vi "SR860 Ramp DC+AC Voltage.vi"() -> ()   [LabVIEW 2025]
doc: "VI to ramp DC Offset of SR860/865 Lockin over time. AC amplitude is kept constant.\nFor I-V curves\nScott Hannahs NHMFL <sth@magnet.fsu.edu>\nAuthor: Scott Hannahs <sth@magnet.fsu.edu>\n\nThis software is licensed for use under the “MIT License\"\nCopyright (c) 2025 Scott Hannahs, sth@sth@magnet.sthnet.net\n\nPermission is hereby granted, free of charge, to any person obtaining a copy of this software and associated documentation files (the \"Software\"), to deal in the Software without restriction, including without limitation the rights to use, copy, modify, merge, publish, distribute, sublicense, and/or sell copies of the Software, and to permit persons to whom the Software is furnished to do so, subject to the following conditions: The above copyright notice and this permission notice shall be included in all copies or substantial portions of the Software.\n\nTHE SOFTWARE IS PROVIDED \"AS IS\", WITHOUT WARRANTY OF ANY KIND, EXPRESS OR IMPLIED, INCLUDING BUT NOT LIMITED TO THE WARRANTIES OF MERCHANTABILITY, FITNESS FOR A PARTICULAR PURPOSE AND NONINFRINGEMENT. IN NO EVENT SHALL THE AUTHORS OR COPYRIGHT HOLDERS BE LIABLE FOR ANY CLAIM, DAMAGES OR OTHER LIABILITY, WHETHER IN AN ACTION OF CONTRACT, TORT OR OTHERWISE, ARISING FROM, OUT OF OR IN CONNECTION WITH THE SOFTWARE OR THE USE OR OTHER DEALINGS IN THE SOFTWARE."
panel:
  in  "AC Voltage":dbl=1e-09 min=1e-09 max=2.0 format="%.6g"
  in  "Clone":bool
  out "Time Remaining":dbl=60.0 format="%<%H:%M:%S>t"
  out "DC Output Voltage":dbl format="%_7g"
  in  "Time (Hr:Min:Sec)":dbl=60.0 step=1.0 format="%<%H:%M:%S>t"
  in  "DC Stop Voltage":dbl min=-5.0 max=5.0 format="%.6g"
  in  "Start Ramp":bool
  in  "Update Time":dbl=0.1 format="%.3g"
  in  "stop":bool
  in  "VISA resource name":refnum<visa-resource-name>
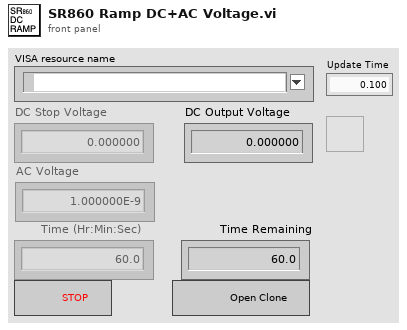
[diagram p1: front panel]
types:
  T1 = enum8{"Enabled", "Disabled", "Disabled and Grayed Out"}
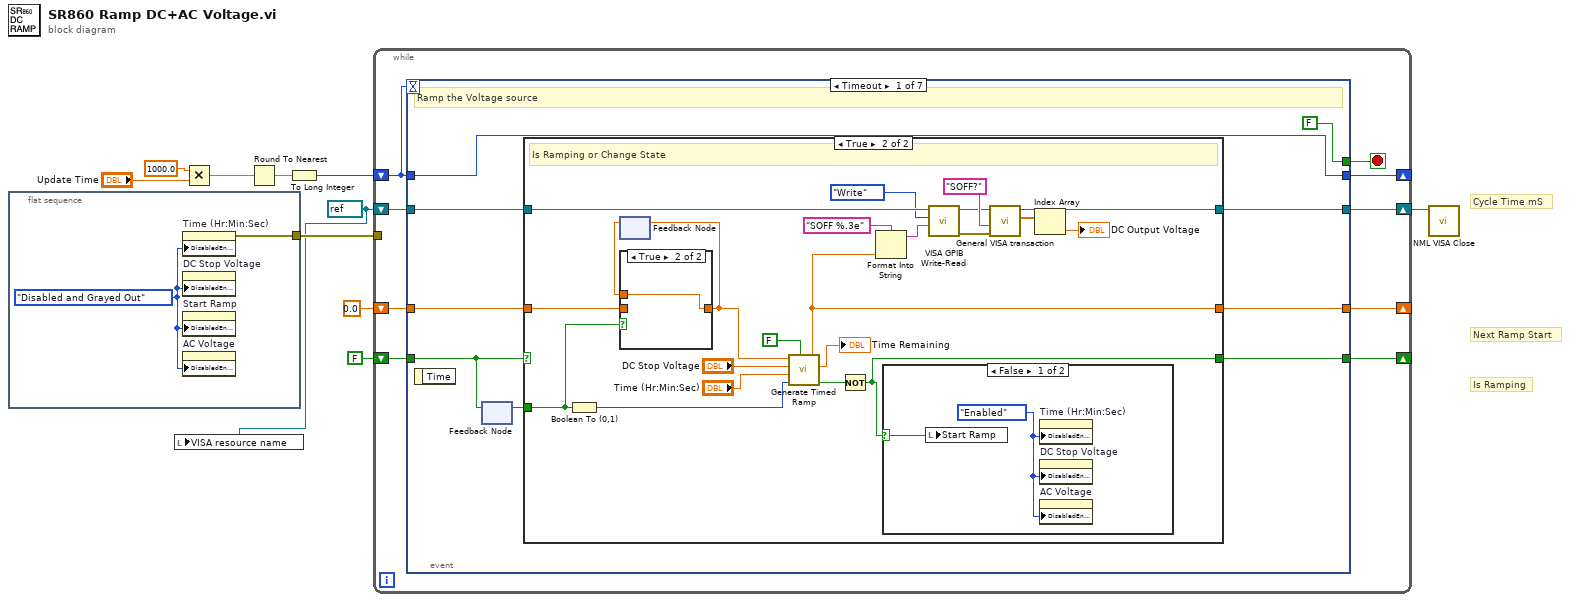
[diagram p0: block diagram]
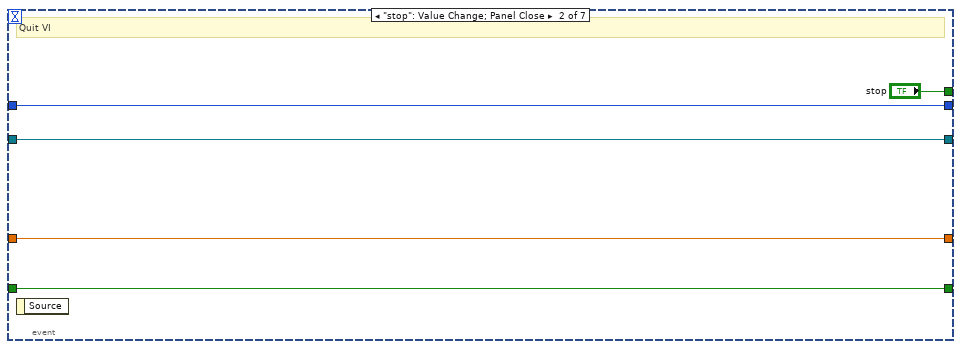
[diagram p5: hidden frame]
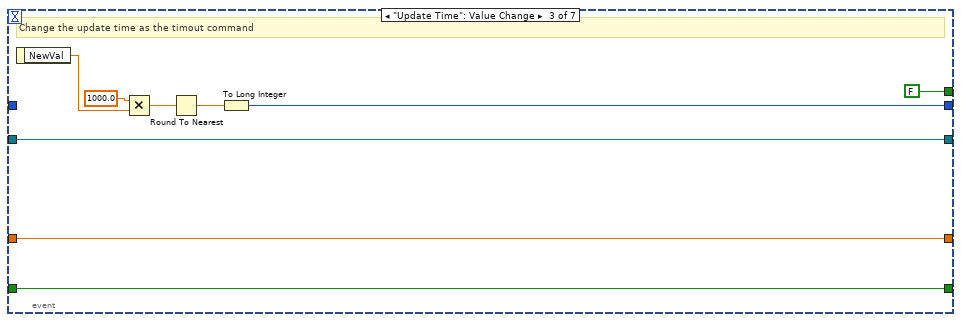
[diagram p6: hidden frame]
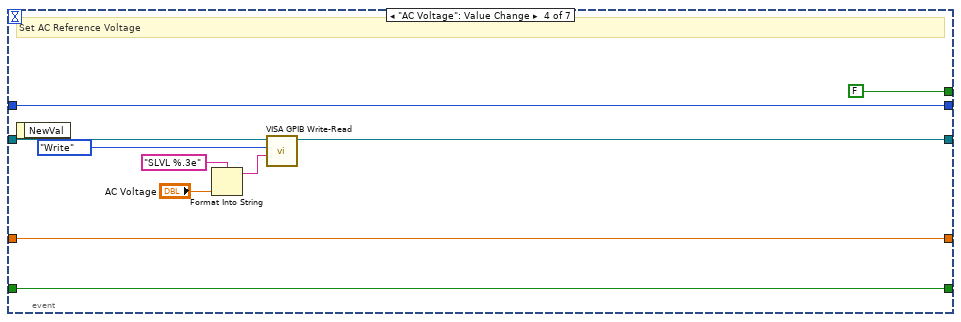
[diagram p7: hidden frame]
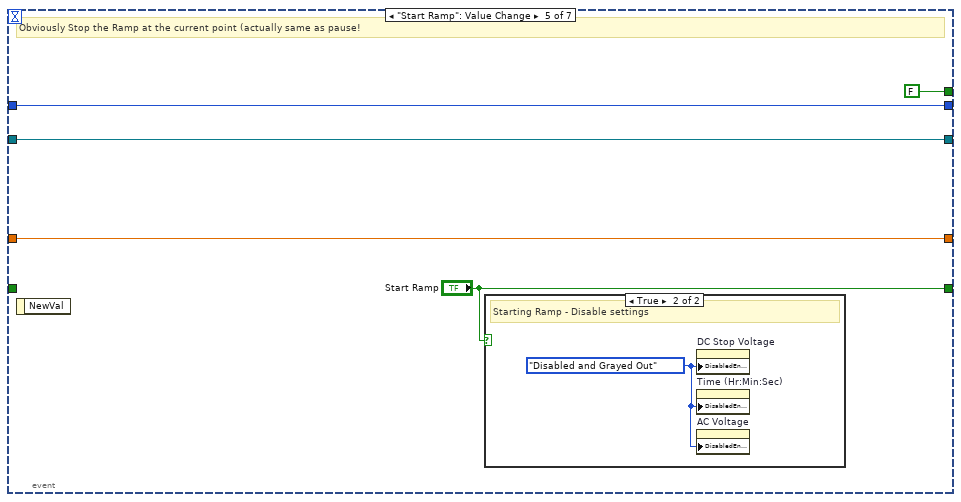
[diagram p8: hidden frame]
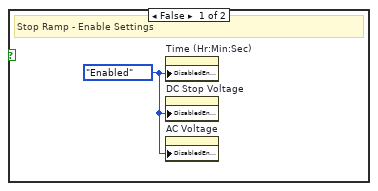
[diagram p9: hidden frame]
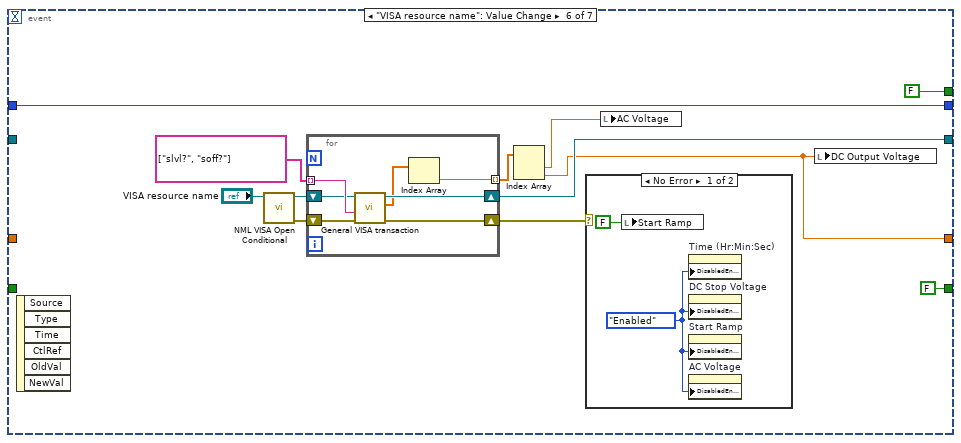
[diagram p10: hidden frame]
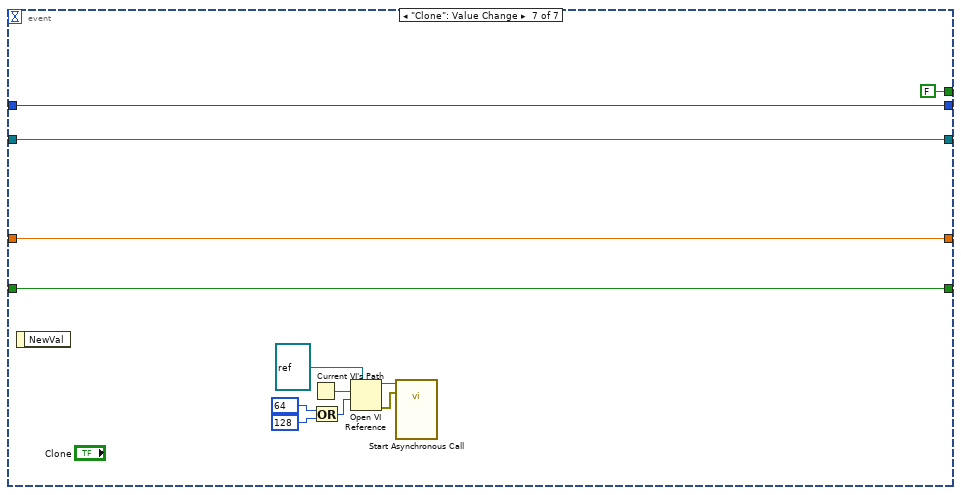
[diagram p12: hidden frame]
diagram:
  w1 = refnum<visa-resource-name> refnum ("dup VISA Session")
  # "Is Ramping"
  # "Next Ramp Start"
  # "Cycle Time mS"
  n1 = flat-sequence {
    tunnel: [w12] -> w2
    frame #0 {
      w11 = T1."Disabled and Grayed Out" ("Disabled")
      n2 = property on="Time (Hr:Min:Sec)" class="DigNum (strict)"("DisabledEnum"=w11) -> (error out=w12:errorcluster)  [unwired: 2 in, 1 out]
      n3 = property on="DC Stop Voltage" class="DigNum (strict)"("DisabledEnum"=w11) -> ()  [unwired: 2 in, 2 out]
      n4 = property on="Start Ramp" class="Bool (strict)"("DisabledEnum"=w11) -> ()  [unwired: 2 in, 2 out]
      n5 = property on="AC Voltage" class="DigNum (strict)"("DisabledEnum"=w11) -> ()  [unwired: 2 in, 2 out]
    }
  }
  n6 = local write "VISA resource name"(w1) -> ()
  n7 = Multiply(x=1000.0, y="Update Time") -> (x*y=w9:dbl)
  n8 = Round To Nearest(number=w9) -> (nearest integer value=w7:dbl)
  n9 = To Long Integer(number=w7) -> (32bit integer=w6:i32)
  n10 = while {
    shift-right: [w17] -> w5
    shift-left: w1 -> [w18]
    shift-right: [w14] -> _
    shift-left: 0.0 ("Voitage 2450") -> [w13]
    shift-right: [w19] -> _
    shift-left: w6 -> [w20]
    shift-right: [w15] -> _
    shift-left: FALSE -> [w16]
    tunnel: w2 -> [_]
    stop <- w21 stop-if-true
    n11 = event shown="[0] Timeout" {
      selector: _ -> [_ _ _ _ _ _ _]
      dyn-events: _ -> [_ _ _ _ _ _ _]
      timeout: w20 -> [_ _ _ _ _ _ _]
      tunnel: [FALSE ("stop") "stop" FALSE ("stop") FALSE ("stop") FALSE ("stop") FALSE ("stop") FALSE ("stop")] -> w21
      tunnel: w20 -> [w30 w63 _ w74 w87 w96 w122]
      tunnel: [w30 w63 w69 w74 w87 w96 w122] -> w19
      tunnel: w18 -> [w29 w60 w66 w79 w86 _ w123]
      tunnel: [w28 w60 w66 w78 w86 w100 w123] -> w17
      tunnel: w16 -> [w23 w62 w67 w76 _ _ w119]
      tunnel: [w26 w62 w67 w76 "Start Ramp" FALSE ("Start Ramp") w119] -> w15
      tunnel: [w24 w61 w65 w77 w85 w92 w120] -> w14
      tunnel: w13 -> [w25 w61 w65 w77 w85 _ w120]
      event Timeout {
        # "Ramp the Voltage source"
        n12 = event-data() -> ()  [unwired: 1 in, 1 out]
        n13 = feedback-in #1(w23) -> ()
        n14 = feedback #1() -> (w22:bool)  [unwired: 1 in]
        n15 = case shown="True" w23 {
          selector: w23 -> [w31 _]
          tunnel: w29 -> [w33 w38]
          tunnel: [w33 w39] -> w28
          tunnel: [w31 w50] -> w26
          tunnel: w25 -> [w32 w48]
          tunnel: [w32 w36] -> w24
          tunnel: w22 -> [_ w49]
          frame False {
            # "Idle"
          }
          frame True {
            # "Is Ramping or Change State"
            n16 = Boolean To (0,1)(Boolean=w49) -> (0, 1=w54:i16)
            n17 = feedback #2() -> (w46:dbl)  [unwired: 1 in]
            n18 = case shown="True" w49 {
              tunnel: w48 -> [w56 _]
              tunnel: [w56 w57] -> w47
              tunnel: w46 -> [_ w57]
              frame False {
              }
              frame True {
              }
            }
            n19 = feedback-in #2(w47) -> ()
            n20 = call "Generate Timed Ramp.vi"("Log"=FALSE, "Point #"=w54, "Time (Hr:Min:Sec)"="Time (Hr:Min:Sec)", "Stop"="DC Stop Voltage", "Start"=w47) -> ("Stop"=w53:bool, "Time Remaining"=→"Time Remaining":dbl, "Output"=w36:dbl)  [unwired: 1 out]
            n21 = Not(x=w53) -> (.not. x?=w50:bool)
            n22 = Format Into String(format string="SOFF %.3e", w36) -> (resulting string=w34:string)  [unwired: 2 in, 1 out]
            n23 = case shown="False" w50 {
              selector: w50 -> [w59 _]
              frame False {
                w58 = T1."Enabled" ("Disabled")
                n24 = local write "Start Ramp"(w59) -> ()
                n25 = property on="Time (Hr:Min:Sec)" class="DigNum (strict)"("DisabledEnum"=w58) -> ()  [unwired: 2 in, 2 out]
                n26 = property on="DC Stop Voltage" class="DigNum (strict)"("DisabledEnum"=w58) -> ()  [unwired: 2 in, 2 out]
                n27 = property on="AC Voltage" class="DigNum (strict)"("DisabledEnum"=w58) -> ()  [unwired: 2 in, 2 out]
              }
              frame True {
              }
            }
            n28 = call "VISA GPIB Write-Read.vi"("Command"=w34, "Action"=enum16{"Write", "Read", "Write & Read"}."Write", "VISA resource name"=w38) -> ("error out"=w44:errorcluster, "dup VISA Session"=w40:refnum<visa-resource-name>)  [unwired: 5 in, 2 out]
            n29 = call "General VISA transaction.vi"("error in (no error)"=w44, "Command String"="SOFF?", "VISA Session"=w40) -> ("Measurement"=w43:dbl[], "dup VISA Session"=w39:refnum<visa-resource-name>)  [unwired: 3 in, 4 out]
            n30 = Index Array(array=w43) -> (element=→"DC Output Voltage":dbl)  [unwired: 1 in]
          }
        }
      }
      event "stop": Value Change; Panel Close {
        # "Quit VI"
        n31 = event-data() -> ()  [unwired: 1 in, 1 out]
      }
      event "Update Time": Value Change {
        # "Change the update time as the timout command"
        n32 = event-data() -> ("NewVal"=w70:dbl)  [unwired: 1 in]
        n33 = Multiply(x=1000.0, y=w70) -> (x*y=w71:dbl)
        n34 = Round To Nearest(number=w71) -> (nearest integer value=w73:dbl)
        n35 = To Long Integer(number=w73) -> (32bit integer=w69:i32)
      }
      event "AC Voltage": Value Change {
        # "Set AC Reference Voltage"
        n36 = event-data() -> ()  [unwired: 1 in, 1 out]
        n37 = Format Into String(format string="SLVL %.3e", "AC Voltage") -> (resulting string=w81:string)  [unwired: 2 in, 1 out]
        n38 = call "VISA GPIB Write-Read.vi"("Command"=w81, "Action"=enum16{"Write", "Read", "Write & Read"}."Write", "VISA resource name"=w79) -> ("dup VISA Session"=w78:refnum<visa-resource-name>)  [unwired: 5 in, 3 out]
      }
      event "Start Ramp": Value Change {
        # "Obviously Stop the Ramp at the current point (actually same as pause!"
        n39 = event-data() -> ()  [unwired: 1 in, 1 out]
        n40 = case shown="True" "Start Ramp" {
          frame False {
            w89 = T1."Enabled" ("Disabled")
            # "Stop Ramp - Enable Settings"
            n41 = property on="Time (Hr:Min:Sec)" class="DigNum (strict)"("DisabledEnum"=w89) -> ()  [unwired: 2 in, 2 out]
            n42 = property on="DC Stop Voltage" class="DigNum (strict)"("DisabledEnum"=w89) -> ()  [unwired: 2 in, 2 out]
            n43 = property on="AC Voltage" class="DigNum (strict)"("DisabledEnum"=w89) -> ()  [unwired: 2 in, 2 out]
          }
          frame True {
            w90 = T1."Disabled and Grayed Out" ("Disabled")
            # "Starting Ramp - Disable settings"
            n44 = property on="DC Stop Voltage" class="DigNum (strict)"("DisabledEnum"=w90) -> ()  [unwired: 2 in, 2 out]
            n45 = property on="Time (Hr:Min:Sec)" class="DigNum (strict)"("DisabledEnum"=w90) -> ()  [unwired: 2 in, 2 out]
            n46 = property on="AC Voltage" class="DigNum (strict)"("DisabledEnum"=w90) -> ()  [unwired: 2 in, 2 out]
          }
        }
      }
      event "VISA resource name": Value Change {
        n47 = event-data() -> ()  [unwired: 1 in, 6 out]
        n48 = call "NML VISA Open Conditional.vi"("VISA resource name"="VISA resource name") -> ("error out"=w102:errorcluster, "dup VISA Session"=w99:refnum<visa-resource-name>)  [unwired: 8 in, 1 out]
        n49 = for {
          shift-right: [w109] -> w100
          shift-left: w99 -> [w110]
          shift-right: [w108] -> w101
          shift-left: w102 -> [w107]
          tunnel: string[] ["slvl?", "soff?"] -> [w111] mode=indexing
          tunnel: [w105] -> w93 mode=indexing
          n50 = call "General VISA transaction.vi"("error in (no error)"=w107, "Command String"=w111, "VISA Session"=w110) -> ("error out"=w108:errorcluster, "Measurement"=w106:dbl[], "dup VISA Session"=w109:refnum<visa-resource-name>)  [unwired: 3 in, 3 out]
          n51 = Index Array(array=w106) -> (element=w105:dbl)  [unwired: 1 in]
        }
        n52 = Index Array(array=w93) -> (element #1=w91:dbl, element #2=w92:dbl)  [unwired: 2 in]
        n53 = case shown="No Error" w101 {
          frame No Error {
            w103 = T1."Enabled" ("Disabled")
            n54 = local write "Start Ramp"(FALSE ("Start Ramp")) -> ()
            n55 = property on="Time (Hr:Min:Sec)" class="DigNum (strict)"("DisabledEnum"=w103) -> ()  [unwired: 2 in, 2 out]
            n56 = property on="DC Stop Voltage" class="DigNum (strict)"("DisabledEnum"=w103) -> ()  [unwired: 2 in, 2 out]
            n57 = property on="Start Ramp" class="Bool (strict)"("DisabledEnum"=w103) -> ()  [unwired: 2 in, 2 out]
            n58 = property on="AC Voltage" class="DigNum (strict)"("DisabledEnum"=w103) -> ()  [unwired: 2 in, 2 out]
          }
          frame Error {
          }
        }
        n59 = local write "AC Voltage"(w91) -> ()
        n60 = local write "DC Output Voltage"(w92) -> ()
      }
      event "Clone": Value Change {
        n61 = event-data() -> ()  [unwired: 1 in, 1 out]
        n62 = Current VI's Path() -> (path=w115:path)
        n63 = Or(x=64, y=128) -> (x .or. y?=w112:i32)
        n64 = Open VI Reference(type specifier VI Refnum (for type only)=refnum<vi> refnum, vi path=w115, options=w112) -> (vi reference=w118:refnum<vi>, error out=w117:errorcluster)  [unwired: 3 in]
        n65 = call-by-ref "Start Asynchronous Call"(reference=w118, error in=w117) -> ()  [unwired: 12 in, 2 out]
      }
    }
  }
  n66 = call "NML VISA Close.vi"("VISA resource name"=w5) -> ()  [unwired: 10 in, 1 out]
